vi "fpga pid.vi"() -> ()   [LabVIEW 2025]
uses:
  <vilib>/Platform/TimedLoop/XDataNode/timing_clust.ctl
  <vilib>/Platform/TimedLoop/XDataNode/nitl_modes.ctl
  <vilib>/Platform/TimedLoop/XDataNode/wakeup.ctl
  <vilib>/rvi/IPIntegrationNode/IPINode_Typedef/niFpgaIPINodeSupportedFamilies.ctl
  <vilib>/rvi/Emulation/niFpgaSctlEmulationGetInTimedLoop.vi
  <vilib>/rvi/Emulation/niFpgaEmulationReportErrorSimple.vi
  <vilib>/rvi/Emulation/niFpgaGetClockAttributes.vi
  <vilib>/rvi/Emulation/niFpgaCriticalErrorInLSC.vi
  <vilib>/rvi/IPIntegrationNode/IPINode_Utilities/niFpgaIPINodeSimCore.vi
  <vilib>/platform/TimedLoop/XDataNode/XDataNode.xnode
  <vilib>/rvi/IPIntegrationNode/IPINode_Xnode/niFpgaIPINode.xnode
  PIDSimFiles/xsim.dir/PID_Simple/xsimkC8B3962433E34175BDA3C83AE24154D4.dll
  <vilib>/Platform/TimedLoop/XDataNode/XDNodeRunTimeDep.lvlib
panel:
  in  "ManualControl":fxp<+,32,16> format="%#_21g"
  in  "Reinitialize":bool
  in  "AutoMode":bool=TRUE
  in  "KdCoeff":fxp<+/-,32,8>
  in  "KiCoeff":fxp<+/-,32,8>
  in  "ProportionalGainKc":fxp<+/-,32,8>=1.0
  out "enable":bool
  out "Output":fxp<+,32,16>
  in  "ProcessVariable":fxp<+/-,32,16>
  in  "Setpoint":fxp<+/-,32,16>
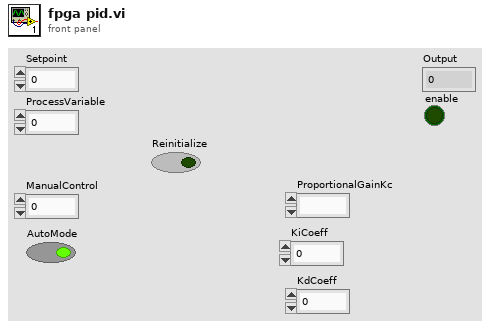
[diagram p1: front panel]
types:
  T1 = typedef "XDNodeRunTimeDep.lvlib/timing_clust.ctl" = cluster{"Expected End [f-1]":u64, "Actual End [f-1]":u64, "Finished Late? [f-1]":bool, "Expected End [i-1]":u64, "Actual End [i-1]":u64, "Finished Late? [i-1]":bool, "Expected Start [i]":u64, "Actual Start [i]":u64, "Expected Start [f]":u64, "Actual Start [f]":u64, "Source Name":string, "Structure Name":string, "Period":i64, "Deadline":i64, "Offset":i64, "Start":i64, "Priority":i32, "Timeout":i32, "Mode":T2, "Wakeup Reason":T3, "Error":errorcluster, "Source Type":string, "Secondary Source Type":string, "Global End Time":u64, "Global Start Time":u64, "Frame Duration":u64, "Iteration Duration":u64, "Assigned CPU":i32, "I/O Scan Engine Mode":u32}
  T2 = typedef "XDNodeRunTimeDep.lvlib/nitl_modes.ctl" = enum32{"No Change", "Process missed periods, maintain original phase", "Discard missed periods, maintain original phase", "Process missed periods, ignore original phase", "Discard missed periods, ignore original phase"}
  T3 = typedef "XDNodeRunTimeDep.lvlib/wakeup.ctl" = enum32{"Normal", "Aborted", "Asynchronous wakeup", "Timing source error", "Timed loop error", "Timeout"}
  T4 = typedef "niFpgaIPINodeSupportedFamilies.ctl" = cluster{"unlimited?":bool, "supported targets":string[]}
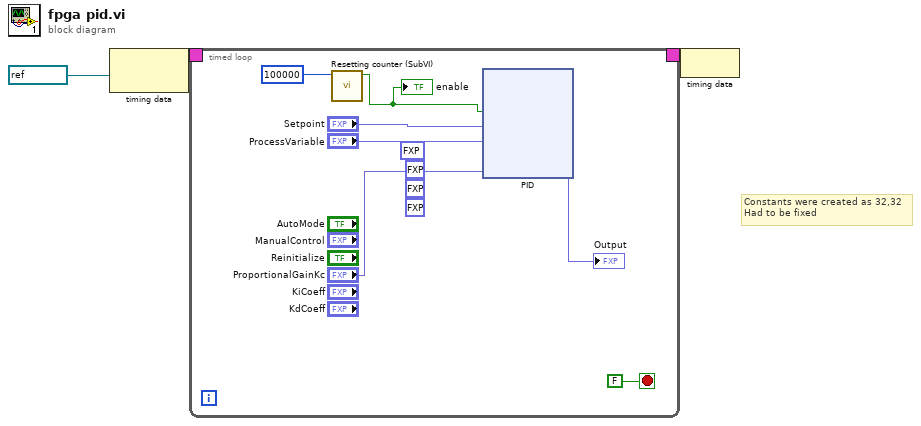
[diagram p0: block diagram]
diagram:
  # "Constants were created as 32,32\nHad to be fixed"
  n1 = node-c288(refnum<k21> "5MHz" ("Source Name")) -> (w3:T1)
  n2 = timed-loop {
    timing: w3 -> [_]
    timing-out: [_] -> w2
    stop <- FALSE stop-if-true
    (unwired) fxp<+/-,32,16> 0.0 ("OutputLow")
    (unwired) fxp<+/-,32,16> 10.0 ("OutputHigh")
    (unwired) fxp<+/-,32,16> 0.0 ("SetpointLow")
    (unwired) fxp<+/-,32,16> 100.0 ("SetpointHigh")
    n3 = call "Resetting counter (SubVI).vi"("Numeric"=u64 100000) -> ("Boolean"=w5:bool)  [unwired: 10 in]
    "enable" <- w5
    n4 = xnode ("PID")("Ce"=w5, "Setpoint"="Setpoint", "ProcessVariable"="ProcessVariable", "ProportionalGainKp"="ProportionalGainKc") -> ("Output"=→"Output":fxp<+,32,16>)
  }
  n5 = node-c288(w2) -> ()
